vi "xiC - IMAQ - Globals.vi"() -> ()   [LabVIEW 2018]
uses:
  xiC - IMAQ - Attributes.ctl
  D:/codes labview/VisionLibrariesXimea/xiLib/xiLIB_64bit/xiLIB/xiCamLib/API/x64/xiApi.NETX64.dll
  xiCamLib/API/x64/xiApi.NETX64.dll
  xiC - IMAQ - TreeDisplayType.ctl
  xiCamLib/xiLIB/Typedefs/xiLIB - Device_Type.ctl
panel:
  in  "Active_xiDeviceType":T1=enum."PCIe"
  in  "ERROR TEXT":string
  in  "Attributes":T2
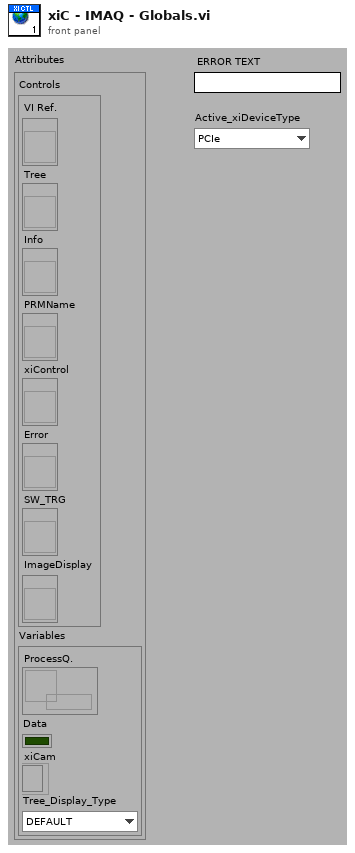
[diagram p1: front panel]
types:
  T1 = typedef "xiLIB - Device_Type.ctl" = enum16{"USB2.0", "USB3.0", "CURRERA", "PCIe", "1394"}
  T2 = typedef "xiC - IMAQ - Attributes.ctl" = cluster{"Controls":cluster{"VI Ref.":refnum<vi>, "Tree":refnum<vi>, "Info":refnum<vi>, "PRMName":refnum<vi>, "xiControl":refnum<vi>, "Error":refnum<vi>, "SW_TRG":refnum<vi>, "ImageDisplay":refnum<vi>}, "Variables":cluster{"ProcessQ.":refnum<queue>, "Data":bool, "xiCam":refnum<k24>, "Tree_Display_Type":T3}}
  T3 = typedef "xiC - IMAQ - TreeDisplayType.ctl" = enum16{"DEFAULT", "HIDE_MAX_MIN"}
diagram:
